vi "SettingsGFV.vi"(8 "error in (no error)":errorcluster, 10 "Variant Input":variant, 11 "Enum":T1=enum."Get Ramp Path") -> (0 "error out":errorcluster, 3 "Variant Output":variant)   [LabVIEW 2013]
doc: "Use this template to build a VI to use as a subVI."
uses:
  SettingsEnum.ctl
  SettingsDataCluster.ctl
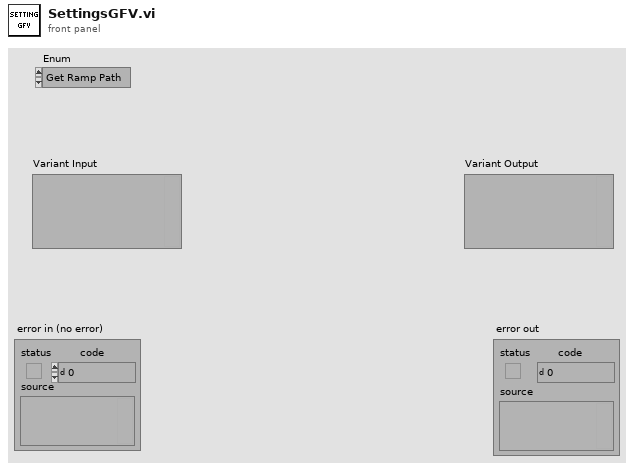
[diagram p1: front panel]
types:
  T1 = typedef "SettingsEnum.ctl" = enum16{"Set Ramp Path", "Set Main Path", "Get Ramp Path", "Set All Data", "Get Main Path", "Init"}
  T2 = typedef "SettingsDataCluster.ctl" = cluster{"Main Path":path, "Ramp Path":path}
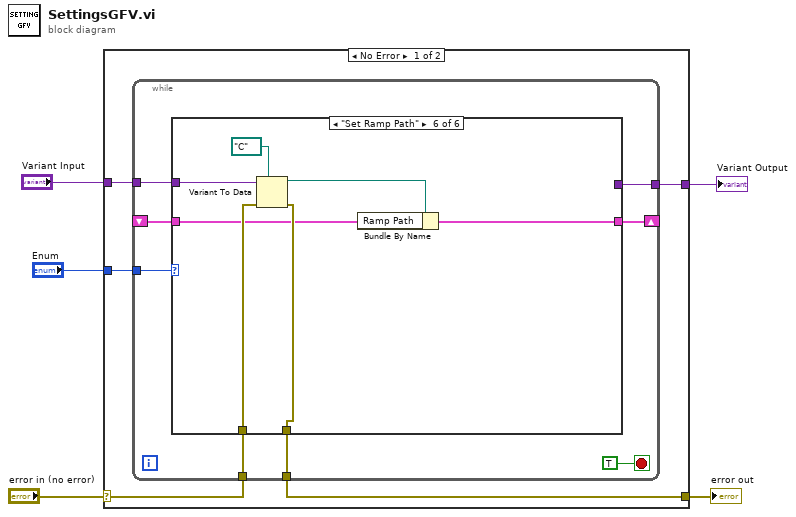
[diagram p0: block diagram]
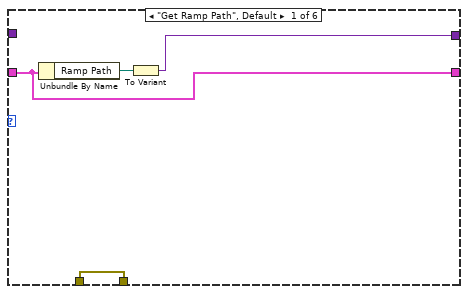
[diagram p2: hidden frame]
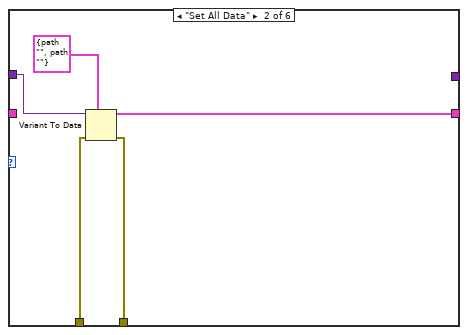
[diagram p3: hidden frame]
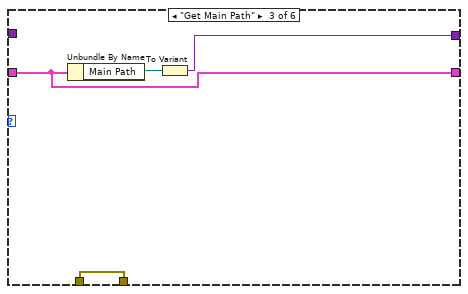
[diagram p4: hidden frame]
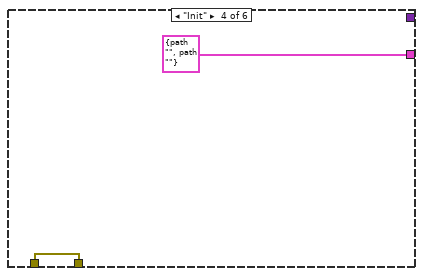
[diagram p5: hidden frame]
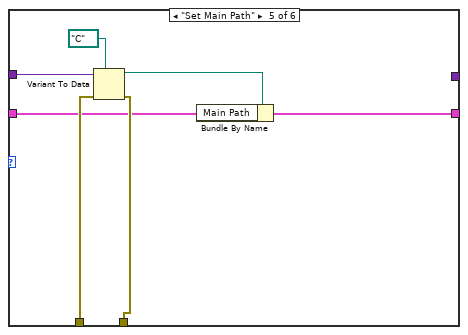
[diagram p6: hidden frame]
diagram:
  n1 = case shown="No Error" "error in (no error)" {
    selector: "error in (no error)" -> [w8 w48]
    tunnel: [w7 w48] -> w4
    tunnel: "Enum" -> [w10 _]
    tunnel: "Variant Input" -> [w9 _]
    tunnel: [w6 _] -> w1
    frame No Error {
      n2 = while {
        tunnel: w10 -> [w17]
        tunnel: w9 -> [w16]
        shift-right: [w15] -> _
        shift-left: _ -> [w12]
        tunnel: w8 -> [w14]
        tunnel: [w13] -> w7
        tunnel: [w11] -> w6
        stop <- TRUE stop-if-true
        n3 = case shown="\"Set Ramp Path\"" w17 {
          tunnel: w16 -> [_ w27 _ _ w40 w47]
          tunnel: [w20 w25 w29 T2 {"Main Path"=path "", "Ramp Path"=path ""} w34 w41] -> w15
          tunnel: w14 -> [w21 w24 w28 w32 w39 w46]
          tunnel: [w21 w23 w28 w32 w38 w45] -> w13
          tunnel: w12 -> [w20 _ w29 _ w36 w43]
          tunnel: [w19 _ w30 _ _ _] -> w11
          frame "Get Ramp Path", Default {
            n4 = Unbundle By Name(w20) -> ("Ramp Path"=w22:path)
            n5 = To Variant(anything=w22) -> (Variant=w19:variant)
          }
          frame "Set All Data" {
            n6 = Variant To Data(error in=w24, type=T2 {"Main Path"=path "", "Ramp Path"=path ""}, Variant=w27) -> (data=w25:T2, error out=w23:errorcluster)
          }
          frame "Get Main Path" {
            n7 = Unbundle By Name(w29) -> ("Main Path"=w31:path)
            n8 = To Variant(anything=w31) -> (Variant=w30:variant)
          }
          frame "Init" {
          }
          frame "Set Main Path" {
            n9 = Variant To Data(error in=w39, type=path "C:/" ("default value"), Variant=w40) -> (data=w35:path, error out=w38:errorcluster)
            n10 = Bundle By Name(cluster=w36, "Main Path"=w35) -> (w34:T2)
          }
          frame "Set Ramp Path" {
            n11 = Variant To Data(error in=w46, type=path "C:/" ("default value"), Variant=w47) -> (data=w42:path, error out=w45:errorcluster)
            n12 = Bundle By Name(cluster=w43, "Ramp Path"=w42) -> (w41:T2)
          }
        }
      }
    }
    frame Error {
    }
  }
  "error out" <- w4
  "Variant Output" <- w1
